vi "Calculate Battery.vi"(11 "Battery A/D in":dbl) -> (3 "Battery Volts Out":dbl)   [LabVIEW 2015]
uses:
  Controls/Gen2 FT Globals.vi
  <vilib>/gmath/NI_Gmath.lvlib
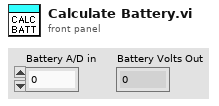
[diagram p1: front panel]
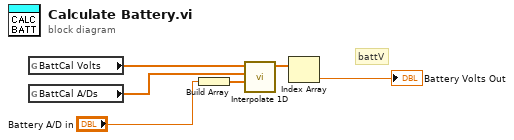
[diagram p0: block diagram]
diagram:
  # "battV"
  n1 = global read "Gen2 FT Globals.vi" "BattCal Volts"() -> (w2:dbl[])
  n2 = global read "Gen2 FT Globals.vi" "BattCal A/Ds"() -> (w1:dbl[])
  n3 = Build Array("Battery A/D in") -> (w5:dbl[])
  n4 = call <vilib>:"Interpolate 1D.vi"("xi"=w5, "X"=w1, "Y"=w2) -> ("yi"=w4:dbl[])  [unwired: 6 in, 2 out]
  n5 = Index Array(array=w4) -> (element=→"Battery Volts Out":dbl)  [unwired: 1 in]
